vi "Draw Crosshair.vi"(7 "Color":u32, 8 "error in (no error)":errorcluster, 9 "Y":i32, 10 "X":i32, 11 "Refnum in":T1) -> (0 "error out":errorcluster, 3 "Refnum out":T1)   [LabVIEW 2016]
uses:
  <vilib>/vision/Image Controls.llb/IMAQ Image.ctl
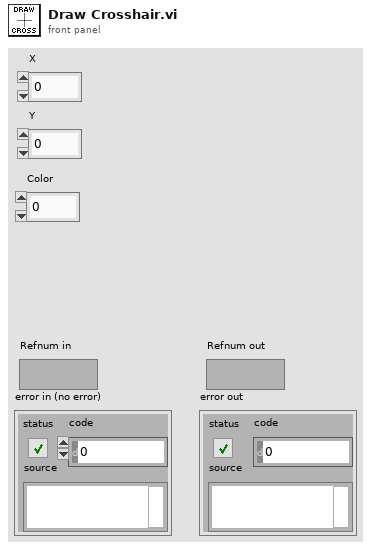
[diagram p1: front panel]
types:
  T1 = typedef "IMAQ Image.ctl" = refnum<image>
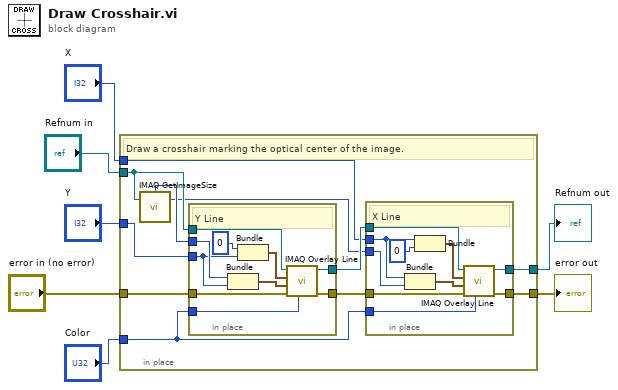
[diagram p0: block diagram]
diagram:
  n1 = in-place {
    in-place-border: "Refnum in" -> [w10]
    in-place-border: [w16] -> w4
    in-place-border: "error in (no error)" -> [w15]
    in-place-border: [w14] -> w3
    in-place-border: "Color" -> [w13]
    in-place-border: "X" -> [w12]
    in-place-border: "Y" -> [w11]
    # "Draw a crosshair marking the optical center of the image."
    n2 = call "IMAQ GetImageSize"("Image"=w10) -> ("Y Resolution"=w8:i32, "X Resolution"=w9:i32)  [unwired: 3 in, 1 out]
    n3 = in-place {
      in-place-border: [w25] -> w18
      in-place-border: [w24] -> w17
      in-place-border: w15 -> [w20]
      in-place-border: w10 -> [w23]
      in-place-border: w9 -> [w22]
      in-place-border: w11 -> [w21]
      in-place-border: w13 -> [w19]
      # "Y Line"
      n4 = Bundle("X Resolution"=w22, "Y"=w21) -> (w26:cluster{"X Resolution":i32, "Y":i32})  [unwired: 1 in]
      n5 = Bundle(0, "Y"=w21) -> (w27:cluster{i32, "Y":i32})  [unwired: 1 in]
      n6 = call "IMAQ Overlay Line"("Color"=w19, "error in (no error)"=w20, "End Point"=w26, "Start Point"=w27, "Image"=w23) -> ("error out"=w24:errorcluster, "Image Out"=w25:T1)  [unwired: 5 in]
    }
    n7 = in-place {
      in-place-border: w18 -> [w37]
      in-place-border: [w34] -> w14
      in-place-border: w17 -> [w33]
      in-place-border: [w32] -> w16
      in-place-border: w12 -> [w31]
      in-place-border: w8 -> [w30]
      in-place-border: w13 -> [w29]
      # "X Line"
      n8 = Bundle("X"=w31, "Y Resolution"=w30) -> (w35:cluster{"X":i32, "Y Resolution":i32})  [unwired: 1 in]
      n9 = Bundle("X"=w31, 0) -> (w36:cluster{"X":i32, i32})  [unwired: 1 in]
      n10 = call "IMAQ Overlay Line"("Color"=w29, "error in (no error)"=w33, "End Point"=w35, "Start Point"=w36, "Image"=w37) -> ("error out"=w32:errorcluster, "Image Out"=w34:T1)  [unwired: 5 in]
    }
  }
  "error out" <- w4
  "Refnum out" <- w3
